vi "Generate_Bivariate_Ranges.vi"(8 "Range mean SD Y":T2={"Size"=30.0, "Min"=0.1, "Max/Step"=0.1, "Max (T) / Step (F)"=FALSE}, 9 "Range mean SD X":T2={"Size"=30.0, "Min"=0.1, "Max/Step"=0.1, "Max (T) / Step (F)"=FALSE}, 10 "Range mean Y":T2={"Size"=39.0, "Min"=1.0, "Max/Step"=0.5, "Max (T) / Step (F)"=FALSE}, 11 "Range mean X":T2={"Size"=18.0, "Min"=3.0, "Max/Step"=1.0, "Max (T) / Step (F)"=FALSE}) -> (0 "Range SD B":dbl[](array[numeric]), 1 "Range SD A":dbl[](array[numeric]), 2 "Range Mean B":dbl[](array[numeric]), 3 "Range Mean A":dbl[](array[numeric]), 4 "N Calculations":i32, 6 "output cluster":T1)   [LabVIEW 2017]
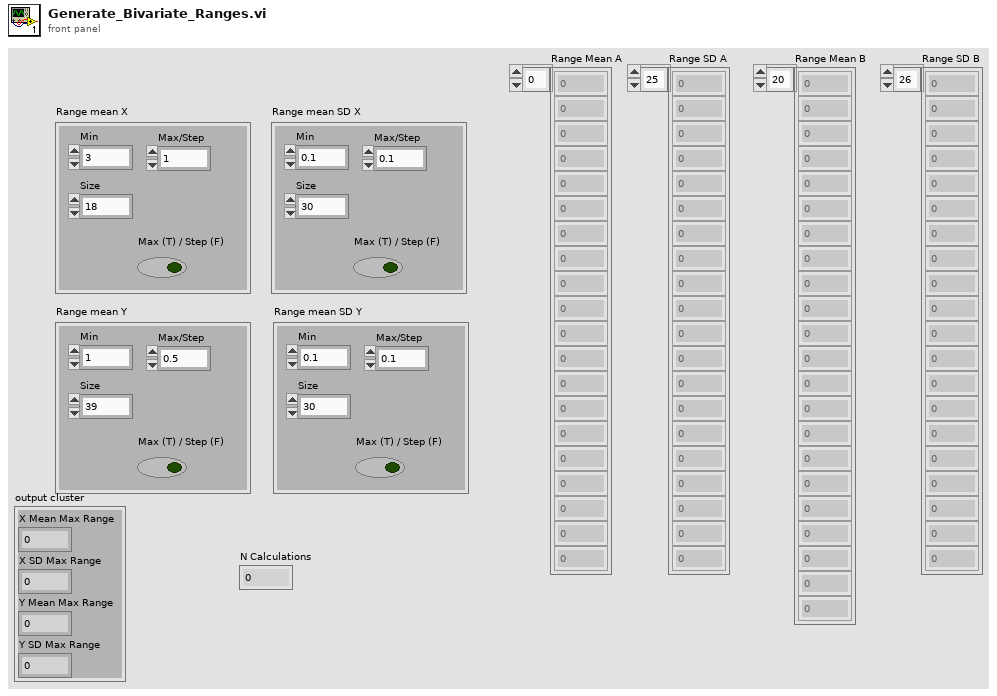
[diagram p1: front panel]
types:
  T1 = cluster{"X Mean Max Range":dbl, "X SD Max Range":dbl, "Y Mean Max Range":dbl, "Y SD Max Range":dbl}
  T2 = cluster{"Size":dbl, "Min":dbl, "Max/Step":dbl, "Max (T) / Step (F)":bool}
  T3 = cluster{"Max Range":dbl, "Max Range":dbl, "Max Range":dbl, "Max Range":dbl}
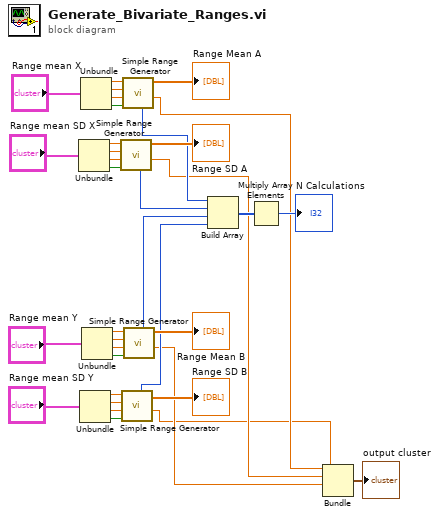
[diagram p0: block diagram]
diagram:
  n1 = Unbundle("Range mean SD X") -> ("Size"=w16:dbl, "Min"=w30:dbl, "Max/Step"=w29:dbl, "Max (T) / Step (F)"=w28:bool)
  n2 = Unbundle("Range mean SD Y") -> ("Size"=w17:dbl, "Min"=w24:dbl, "Max/Step"=w23:dbl, "Max (T) / Step (F)"=w22:bool)
  n3 = Unbundle("Range mean X") -> ("Size"=w34:dbl, "Min"=w33:dbl, "Max/Step"=w32:dbl, "Max (T) / Step (F)"=w31:bool)
  n4 = Unbundle("Range mean Y") -> ("Size"=w18:dbl, "Min"=w27:dbl, "Max/Step"=w26:dbl, "Max (T) / Step (F)"=w25:bool)
  n5 = call "Simple Range Generator.vi"("Size"=w16, "Min"=w30, "Max/Step"=w29, "Max (T) / Step (F)"=w28) -> ("N Calculations"=w10:i32, "Array"=→"Range SD A":dbl[], "Max Range"=w4:dbl)  [unwired: 2 out]
  n6 = call "Simple Range Generator.vi"("Size"=w17, "Min"=w24, "Max/Step"=w23, "Max (T) / Step (F)"=w22) -> ("N Calculations"=w8:i32, "Array"=→"Range SD B":dbl[], "Max Range"=w2:dbl)  [unwired: 2 out]
  n7 = call "Simple Range Generator.vi"("Size"=w34, "Min"=w33, "Max/Step"=w32, "Max (T) / Step (F)"=w31) -> ("N Calculations"=w11:i32, "Array"=→"Range Mean A":dbl[], "Max Range"=w5:dbl)  [unwired: 2 out]
  n8 = call "Simple Range Generator.vi"("Size"=w18, "Min"=w27, "Max/Step"=w26, "Max (T) / Step (F)"=w25) -> ("N Calculations"=w9:i32, "Array"=→"Range Mean B":dbl[], "Max Range"=w3:dbl)  [unwired: 2 out]
  n9 = Build Array(w11, w10, w9, w8) -> (w7:i32[])
  n10 = Multiply Array Elements(1:w7) -> (0:→"N Calculations":i32)
  n11 = Bundle("Max Range"=w5, "Max Range"=w4, "Max Range"=w3, "Max Range"=w2) -> (→"output cluster":T3)  [unwired: 1 in]
